vi "Get LabVIEW Data Directory.vi"(8 "Error In":errorcluster) -> (0 "Error Out":errorcluster, 2 "LabVIEW Data Path":string)   [LabVIEW 2014, in "LMH-Toolbox.lvlib"]
doc: "This VI returns the LabVIEW Data Directory. For example:\n\nC:\\Users\\LabVIEW Hacker\\Documents\\LabVIEW Data"
uses:
  <vilib>/MakerHub/Toolbox/LMH-Toolbox.lvlib
  <vilib>/registry/registry.llb/Registry RtKey.ctl
  <vilib>/registry/registry.llb/Read Registry Value Simple.vi
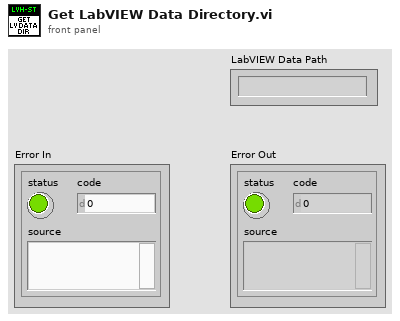
[diagram p1: front panel]
types:
  T1 = typedef "Registry RtKey.ctl" = enum32{"HKEY_CLASSES_ROOT", "HKEY_CURRENT_USER", "HKEY_LOCAL_MACHINE", "HKEY_USERS", "HKEY_PERFORMANCE_DATA", "HKEY_CURRENT_CONFIG", "HKEY_DYN_DATA"}
  T2 = typedef "Registry refnum.ctl" = refnum<k1>
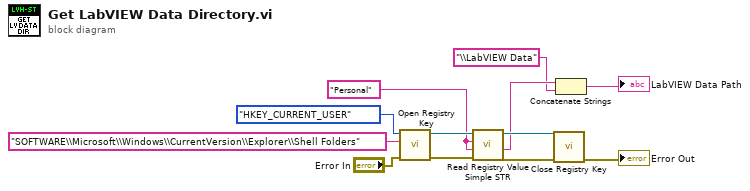
[diagram p0: block diagram]
diagram:
  w6 = "Personal"
  n1 = call <vilib>:"Open Registry Key.vi"("error in (no error)"="Error In", "subkey"="SOFTWARE\\Microsoft\\Windows\\CurrentVersion\\Explorer\\Shell Folders", "root key (HKEY_LOCAL_MACHINE)"=Registry_RtKey."HKEY_CURRENT_USER") -> ("error out"=w10:errorcluster, "refnum out"=w9:T2)  [unwired: 7 in]
  n2 = call-poly <vilib>:"Read Registry Value Simple STR.vi"("error in (no error)"=w10, "default data"=w6, "value"=w6, "refnum"=w9) -> ("error out"=w7:errorcluster, "String/Binary data"=w5:string, "refnum out"=w8:T2)  [unwired: 2 in, 1 out]
  n3 = call <vilib>:"Close Registry Key.vi"("error in (no error)"=w7, "refnum"=w8) -> ("error out"=→"Error Out":errorcluster)  [unwired: 5 in]
  n4 = Concatenate Strings(w5, "\\LabVIEW Data" ("string")) -> (→"LabVIEW Data Path":string)
